vi "PID.vi"(9 "Sensor Derivative":dbl, 10 "Servo Params":T1, 11 "Error":dbl) -> (3 "Out":dbl)   [LabVIEW 2016]
uses:
  <vilib>/Rock Robotics/WPI/ThirdParty/CanMotor/CTRLib-LV-TalonSRX/Framework/ServoParams.ctl
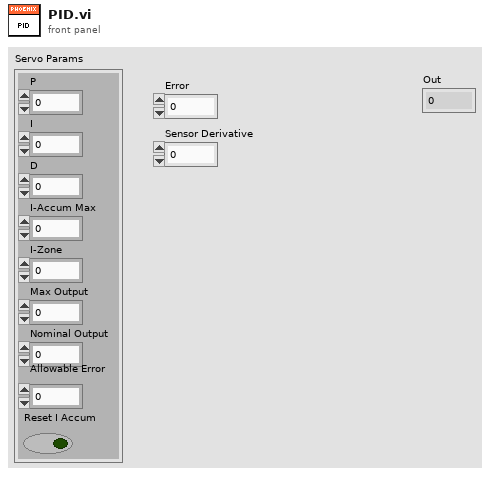
[diagram p1: front panel]
types:
  T1 = typedef "ServoParams.ctl" = cluster{"P":dbl, "I":dbl, "D":dbl, "I-Accum Max":dbl, "I-Zone":dbl, "Max Output":dbl, "Nominal Output":dbl, "Allowable Error":dbl, "Reset I Accum":bool}
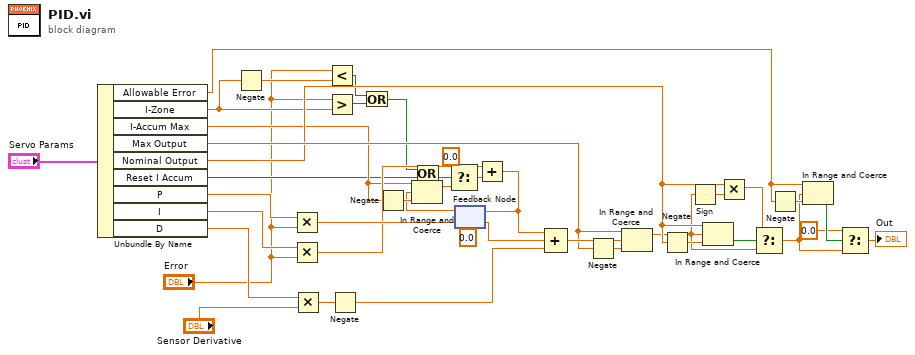
[diagram p0: block diagram]
diagram:
  n1 = Unbundle By Name("Servo Params") -> ("Allowable Error"=w5:dbl, "I-Zone"=w12:dbl, "I-Accum Max"=w18:dbl, "Max Output"=w27:dbl, "Nominal Output"=w24:dbl, "Reset I Accum"=w15:bool, "P"=w37:dbl, "I"=w36:dbl, "D"=w32:dbl)
  n2 = Negate(x=w12) -> (-x=w11:dbl)
  n3 = Multiply(x=w37, y="Error") -> (x*y=w35:dbl)
  n4 = Multiply(x=w36, y="Error") -> (x*y=w34:dbl)
  n5 = Multiply(x=w32, y="Sensor Derivative") -> (x*y=w14:dbl)
  n6 = Less?(x="Error", y=w11) -> (x < y?=w8:bool)
  n7 = Greater?(x="Error", y=w12) -> (0:w9:bool)
  n8 = Negate(x=w14) -> (-x=w13:dbl)
  n9 = Or(x=w8, y=w9) -> (x .or. y?=w7:bool)
  n10 = Negate(x=w18) -> (-x=w20:dbl)
  n11 = Or(x=w7, y=w15) -> (x .or. y?=w16:bool)
  n12 = feedback #1(0.0) -> (w17:dbl)
  n13 = In Range and Coerce(upper limit=w18, x=w17, lower limit=w20) -> (coerced(x)=w19:dbl)  [unwired: 1 out]
  n14 = Select(t=0.0, s=w16, f=w19) -> (s? t:f=w31:dbl)
  n15 = Add(x=w34, y=w31) -> (x+y=w40:dbl)
  n16 = feedback-in #1(w40) -> ()
  n17 = Compound Arithmetic op=ADD(w40, w35, w13) -> (w29:dbl)
  n18 = Negate(x=w27) -> (-x=w28:dbl)
  n19 = In Range and Coerce(upper limit=w27, x=w29, lower limit=w28) -> (coerced(x)=w22:dbl)  [unwired: 1 out]
  n20 = Negate(x=w24) -> (-x=w26:dbl)
  n21 = Sign(1:w22) -> (0:w23:dbl)
  n22 = In Range and Coerce(upper limit=w24, x=w22, lower limit=w26) -> (In Range?=w25:bool)  [unwired: 1 out]
  n23 = Multiply(x=w24, y=w23) -> (x*y=w21:dbl)
  n24 = Select(t=w21, s=w25, f=w22) -> (s? t:f=w2:dbl)
  n25 = Negate(x=w5) -> (-x=w6:dbl)
  n26 = In Range and Coerce(upper limit=w5, x=w2, lower limit=w6) -> (In Range?=w3:bool)  [unwired: 1 out]
  n27 = Select(t=0.0, s=w3, f=w2) -> (s? t:f=→"Out":dbl)
